vi "取出力曲线C.vi"(2 "cPr":T1={"选择"=enum."Fx", "系数x"=1.0, "系数+"=1.0, "上限"=4.3, "下限"=3.7, "Ymax"=50.0, "Ymin"=-50.0, "点数"=1000.0, "锁系数x"=1.0, "锁上限"=0.4, "锁下限"=0.6, "锁系数+"=1.0, "起点"=0.20000000298023224, "终点"=0.6499999761581421, "锁起点"=0.05000000074505806, "锁终点"=0.20000000298023224, "上参考"=4.3, "下参考"=3.7, "基准"=3.7} {"系数+" format="%.3f"; "基准" format="%.2f"; "下参考" format="%.2f"; "上参考" format="%.2f"; "锁终点" format="%.2f"; "锁起点" format="%.2f"; "终点" format="%.2f"; "起点" format="%.2f"; "锁系数+" format="%.3f"; "锁下限" format="%.2f"; "锁上限" format="%.2f"; "锁系数x" format="%.3f"; "下限" format="%.2f"; "上限" format="%.2f"; "系数x" format="%.3f"}, 3 "截取?F":bool, 4 "历史数据":T2(array[cluster])) -> (0 "全曲线":sgl[](array[numeric]), 1 "曲线":sgl[](array[numeric]))   [LabVIEW 2018]
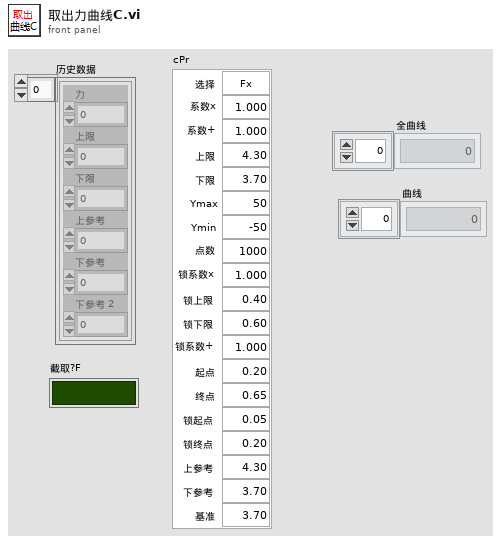
[diagram p1: front panel]
types:
  T1 = cluster{"选择":enum16{"Fx", "Fy", "Fz", "Mx", "My", "Mz"}, "系数x":sgl, "系数+":sgl, "上限":sgl, "下限":sgl, "Ymax":dbl, "Ymin":dbl, "点数":dbl, "锁系数x":sgl, "锁上限":sgl, "锁下限":sgl, "锁系数+":sgl, "起点":dbl, "终点":dbl, "锁起点":dbl, "锁终点":dbl, "上参考":sgl, "下参考":sgl, "基准":sgl}
  T2 = cluster{"力":sgl, "上限":sgl, "下限":sgl, "上参考":sgl, "下参考":sgl, "下参考 2":sgl}[]
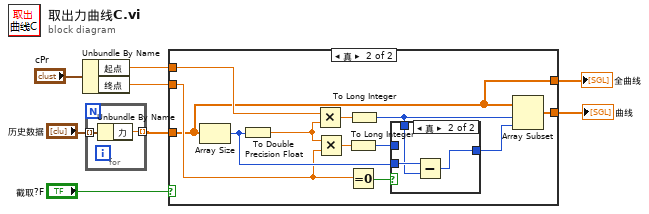
[diagram p0: block diagram]
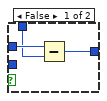
[diagram p3: hidden frame]
diagram:
  n1 = Unbundle By Name("cPr") -> ("起点"=w4:dbl, "终点"=w3:dbl)
  n2 = for {
    tunnel: "历史数据" -> [w10] mode=indexing
    tunnel: [w9] -> w6 mode=indexing
    n3 = Unbundle By Name(w10) -> ("力"=w9:sgl)
  }
  n4 = case shown="真" "截取?F" {
    tunnel: w6 -> [w11 w12]
    tunnel: [w11 w15] -> w5
    tunnel: w4 -> [_ w14]
    tunnel: w3 -> [_ w13]
    tunnel: [w11 w12] -> w2
    frame False {
    }
    frame True {
      n5 = Array Size(array=w12) -> (size(s)=w20:i32)
      n6 = To Double Precision Float(number=w20) -> (double precision float=w16:dbl)
      n7 = Multiply(x=w14, y=w16) -> (x*y=w22:dbl)
      n8 = Multiply(x=w16, y=w13) -> (x*y=w21:dbl)
      n9 = To Long Integer(number=w21) -> (32bit integer=w19:i32)
      n10 = Equal To 0?(x=w13) -> (x = 0?=w23:bool)
      n11 = To Long Integer(number=w22) -> (32bit integer=w18:i32)
      n12 = case shown="真" w23 {
        tunnel: w20 -> [_ w29]
        tunnel: w19 -> [w26 _]
        tunnel: w18 -> [w25 w28]
        tunnel: [w24 w27] -> w17
        frame False {
          n13 = Subtract(x=w26, y=w25) -> (x-y=w24:i32)
        }
        frame True {
          n14 = Subtract(x=w29, y=w28) -> (x-y=w27:i32)
        }
      }
      n15 = Array Subset(array=w12, index=w18, length=w17) -> (w15:sgl[])
    }
  }
  "曲线" <- w5
  "全曲线" <- w2
